vi "DrawTile.vi"(4 "index_y":u16, 5 "Tilebuffer":refnum<k21>="TileBuffer", 6 "index_x":u16, 7 "TileNo":u16, 8 "Modifier":u16, 9 "pos_y":u16, 10 "pos_x":u16, 11 "color_in":fxp<+,3,3>) -> (3 "color_out":fxp<+,3,3>)   [LabVIEW 2019, in "Tiles.lvlib"]
uses:
  Tiles.lvlib
  <vilib>/rvi/DataTransferAndStorage/Container/Common/niFpgaContainerExecOnDevCompGetState.vi
  <vilib>/rvi/Emulation/niFpgaEmulationIsFPGAContextNoSignature.vi
  <vilib>/rvi/DataTransferAndStorage/Container/Common/niFpgaContainerGetUniqueNameForEmu.vi
  <vilib>/rvi/Emulation/niFpgaProcessEmulError.vi
  <vilib>/rvi/Emulation/niFpgaSctlEmulationGetInTimedLoop.vi
  <vilib>/rvi/errors/nirviReportUnexpectedCaseInternalError (U32).vi
  <vilib>/rvi/Memory/Memory_Emulation/niFpgaMemoryEmulationCacheClearOnFirstRun.vi
  <vilib>/rvi/Memory/Memory_Emulation/nirvimemoryEmulationManagerCache_MakeExclusive.vi
  <vilib>/rvi/Memory/Memory_Emulation/niFpgaMemoryEmulationValidateCache.vi
  <vilib>/rvi/Memory/Memory_Emulation/nirvimemoryEmulationManagerCache_InsertValue.vi
  <vilib>/Utility/error.llb/Clear Errors.vi
  <vilib>/rvi/Memory/Memory_Emulation/nirvimemoryEmulationManagerCache_ReleaseExclusive.vi
  <vilib>/rvi/Memory/Memory_Emulation/nirvimemoryEmulationManagerCache_GetValue.vi
  <vilib>/rvi/Memory/Memory_Emulation/nirvimemoryEmulationManagerCache_SetValue.vi
  <vilib>/rvi/Emulation/niFpgaSctlEmulationResourceMgr.vi
  <vilib>/rvi/DataTransferAndStorage/Container/XNode/niFpgaContainer.xnode
  <vilib>/rvi/Memory/Memory_Emulation/niFpgaMemoryEmulationRefIn.vi
  GameEngine/GameEngine.lvlib
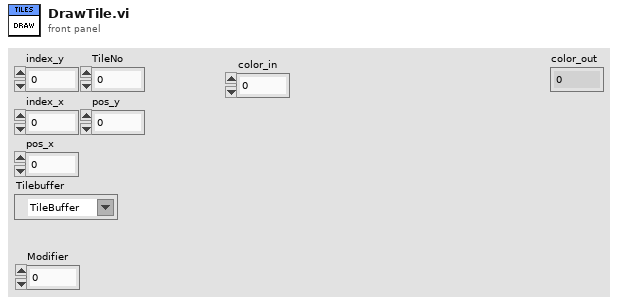
[diagram p1: front panel]
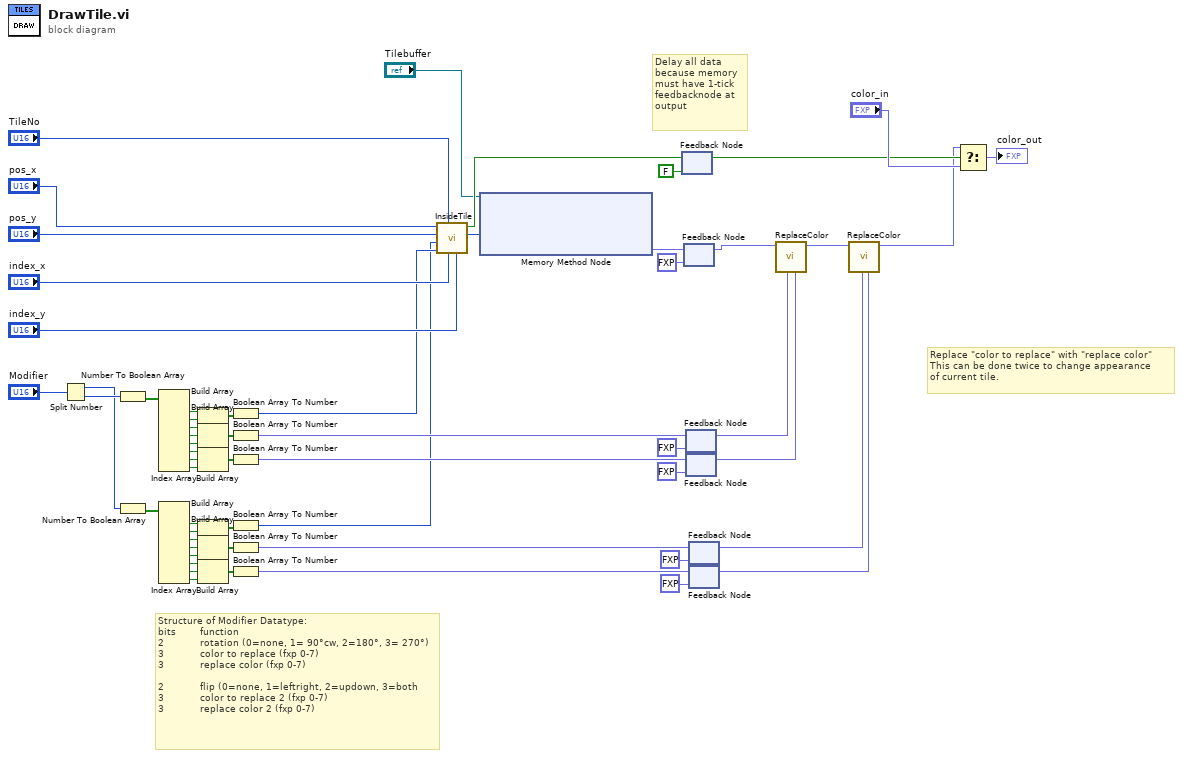
[diagram p0: block diagram]
diagram:
  # "Delay all data\nbecause memory\nmust have 1-tick\nfeedbacknode at\noutput"
  # "Structure of Modifier Datatype:\nbits        function\n2            rotation (0=none, 1= 90°cw, 2=180°, 3= 270°)\n3            color to replace (fxp 0-7)\n3            replace color (fxp 0-7)\n\n2            flip (0=none, 1=leftright, 2=updown, 3=both\n3            color to replace 2 (fxp 0-7)\n3            replace color 2 (fxp 0-7)"
  # "Replace \"color to replace\" with \"replace color\"\nThis can be done twice to change appearance\nof current tile."
  n1 = Split Number(x="Modifier") -> (hi(x)=w15:u8, lo(x)=w43:u8)
  n2 = Number To Boolean Array(number=w43) -> (Boolean array=w42:bool[])
  n3 = Number To Boolean Array(number=w15) -> (Boolean array=w16:bool[])
  n4 = Index Array(array=w42) -> (element #1=w41:bool, element #2=w40:bool, element #3=w39:bool, element #4=w38:bool, element #5=w37:bool, element #6=w36:bool, element #7=w35:bool, element #8=w34:bool)  [unwired: 8 in]
  n5 = Index Array(array=w16) -> (element #1=w17:bool, element #2=w18:bool, element #3=w19:bool, element #4=w20:bool, element #5=w21:bool, element #6=w22:bool, element #7=w23:bool, element #8=w24:bool)  [unwired: 8 in]
  n6 = Build Array(w41, w40) -> (w32:bool[])
  n7 = Build Array(w39, w38, w37) -> (w33:bool[])
  n8 = Build Array(w36, w35, w34) -> (w29:bool[])
  n9 = Build Array(w17, w18) -> (w26:bool[])
  n10 = Build Array(w19, w20, w21) -> (w25:bool[])
  n11 = Build Array(w22, w23, w24) -> (w27:bool[])
  n12 = Boolean Array To Number(Boolean array=w32) -> (number=w31:u8)
  n13 = Boolean Array To Number(Boolean array=w33) -> (number=w30:fxp<+,3,3>)
  n14 = Boolean Array To Number(Boolean array=w29) -> (number=w28:fxp<+,3,3>)
  n15 = Boolean Array To Number(Boolean array=w26) -> (number=w14:u8)
  n16 = Boolean Array To Number(Boolean array=w25) -> (number=w13:fxp<+,3,3>)
  n17 = Boolean Array To Number(Boolean array=w27) -> (number=w11:fxp<+,3,3>)
  n18 = call "InsideTile.vi"("index_y"="index_y", "index_x"="index_x", "TileNo"="TileNo", "rotation"=w31, "flip"=w14, "pos_y"="pos_y", "pos_x"="pos_x") -> ("TilePixelIndex"=w53:u32, "InsideTile?"=w51:bool)  [unwired: 3 in]
  n19 = xnode ("Memory Method Node")("Address"=w53, "Memory In"="Tilebuffer") -> ("Data"=w50:fxp<+,3,3>)  [unwired: 1 out]
  n20 = feedback #1(FALSE ("InsideTile?")) -> (w48:bool)
  n21 = feedback-in #1(w51) -> ()
  n22 = feedback #2(fxp<+,3,3> 0.0 ("Data")) -> (w12:fxp<+,3,3>)
  n23 = feedback-in #2(w50) -> ()
  n24 = feedback-in #3(w30) -> ()
  n25 = feedback #3(fxp<+,3,3> 0.0) -> (w6:fxp<+,3,3>)
  n26 = feedback-in #4(w28) -> ()
  n27 = feedback #4(fxp<+,3,3> 0.0) -> (w5:fxp<+,3,3>)
  n28 = feedback-in #5(w13) -> ()
  n29 = feedback #5(fxp<+,3,3> 0.0) -> (w3:fxp<+,3,3>)
  n30 = feedback-in #6(w11) -> ()
  n31 = feedback #6(fxp<+,3,3> 0.0) -> (w2:fxp<+,3,3>)
  n32 = call "ReplaceColor.vi"("Replace color"=w5, "Color to replace"=w6, "color in"=w12) -> ("color out"=w4:fxp<+,3,3>)  [unwired: 8 in]
  n33 = call "ReplaceColor.vi"("Replace color"=w2, "Color to replace"=w3, "color in"=w4) -> ("color out"=w1:fxp<+,3,3>)  [unwired: 8 in]
  n34 = Select(t=w1, s=w48, f="color_in") -> (s? t:f=→"color_out":fxp<+,3,3>)
